vi "Example 2.vi"() -> ()   [LabVIEW 2019]
uses:
  FINS/FINS_header.ctl
  subvi/Request.ctl
  FINS/FINS CMD.ctl
  FINS/FINS TCP.lvlib
panel:
  out "error":string
  out "CMD":T1
  out "FINS Header Sever":T2={"resp req"=FALSE, "cmd resp"=FALSE, "SID"=255, "DNA"=2, "DA1"=2, "DA2"=2, "SA1"=0, "SA2"=255, "SNA"=255} {"SNA" max=127 format="%x"; "SA2" max=254 step=1 format="%x"; "SA1" format="%x"; "DA2" max=254 step=1 format="%x"; "DA1" format="%x"; "DNA" max=127 step=1 format="%x"}
  out "error TCP out":errorcluster={"status"=TRUE, "code"=56, "source"="TCP Read in main.vi"}
  in  "Request":T3=enum."Read_002"
  out "RSP":bool
  in  "Acces Release":bool
  in  "Acces Acq":bool
  out "t2":dbl
  out "t1":dbl
  out "Client Node":u32=10 format="%x"
  in  "FINS Header Client":T2={"resp req"=TRUE, "cmd resp"=FALSE, "SID"=0, "DNA"=0, "DA1"=10, "DA2"=0, "SA1"=0, "SA2"=251, "SNA"=0} {"SNA" max=127 format="%x"; "SA2" max=254 step=1 format="%x"; "SA1" format="%x"; "DA2" max=254 step=1 format="%x"; "DA1" format="%x"; "DNA" max=127 step=1 format="%x"}
  in  "send request":bool
  out "count":i32=1
  out "Server Node":u32=10 format="%x"
  out "cmd":u32=1
  out "error TCP in":errorcluster={"status"=TRUE, "code"=56, "source"="TCP Read in main.vi"}
  in  "setup":bool
  out "len":i32=24
  out "on":bool
  out "data out":string
  in  "stop":bool=TRUE
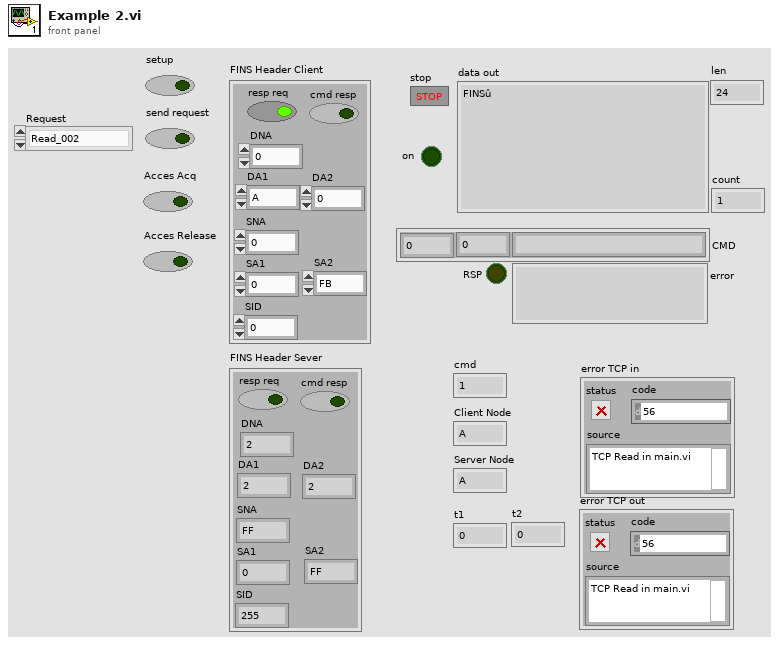
[diagram p1: front panel]
types:
  T1 = typedef "FINS TCP.lvlib/FINS CMD.ctl" = cluster{"MR":u8, "SR":u8, "name":string}
  T2 = typedef "FINS TCP.lvlib/FINS_header.ctl" = cluster{"resp req":bool, "cmd resp":bool, "SID":u8, "DNA":u8, "DA1":u8, "DA2":u8, "SA1":u8, "SA2":u8, "SNA":u8}
  T3 = typedef "Request.ctl" = enum16{"Setup", "Access Right: Acquire", "Access Right: Release", "STOP", "RUN", "Read_001", "Read_002", "Read_003", "Write_001"}
  T4 = enum16{"Standard", "Buffered", "CRLF", "Immediate"}
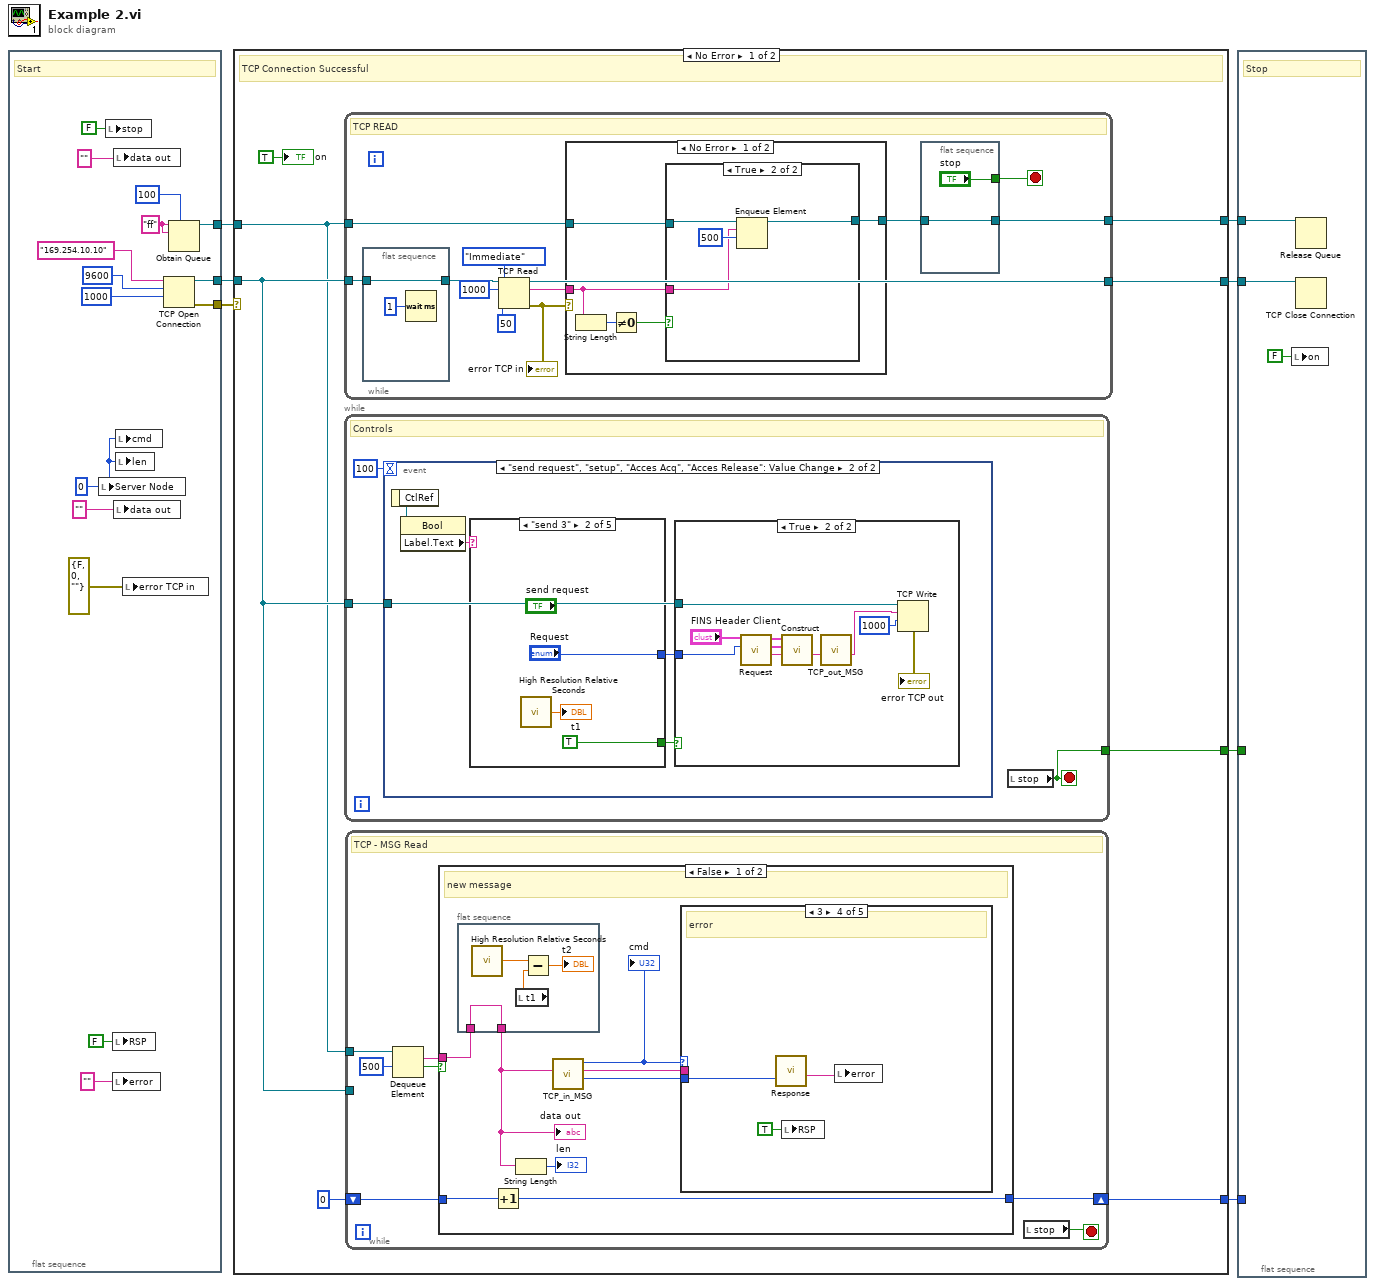
[diagram p0: block diagram]
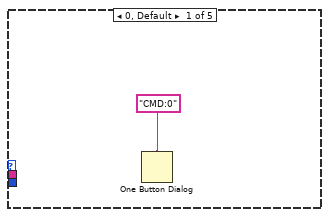
[diagram p2: hidden frame]
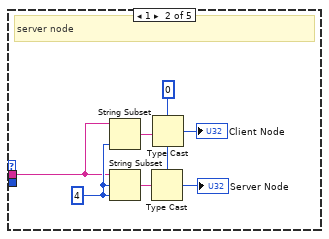
[diagram p3: hidden frame]
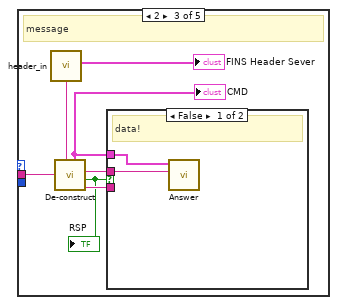
[diagram p4: hidden frame]
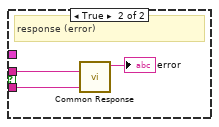
[diagram p5: hidden frame]
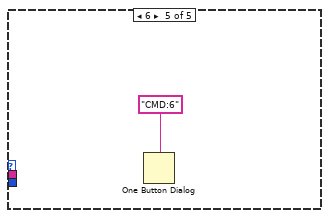
[diagram p6: hidden frame]
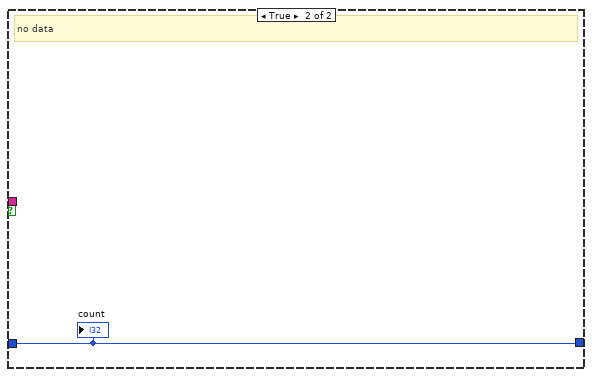
[diagram p7: hidden frame]
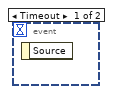
[diagram p8: hidden frame]
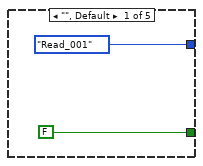
[diagram p10: hidden frame]
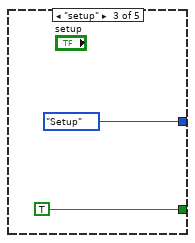
[diagram p11: hidden frame]
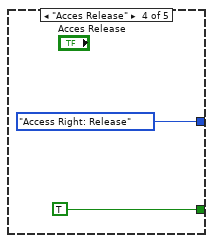
[diagram p12: hidden frame]
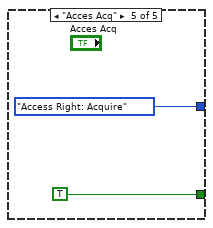
[diagram p13: hidden frame]
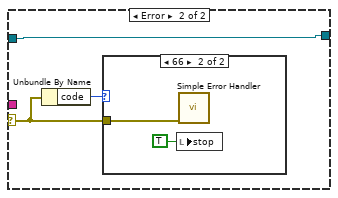
[diagram p15: hidden frame]
diagram:
  n1 = flat-sequence {
    tunnel: [w19] -> w7
    tunnel: [w18] -> w6
    tunnel: [w13] -> w3
    frame #0 {
      w12 = u32 0 ("snode")
      w14 = "ff" ("name (unnamed)")
      # "Start"
      n2 = local write "Server Node"(w12) -> ()
      n3 = local write "stop"(FALSE ("stop")) -> ()
      n4 = local write "RSP"(FALSE ("RSP")) -> ()
      n5 = local write "error"("" ("message")) -> ()
      n6 = local write "data out"("" ("data out")) -> ()
      n7 = local write "data out"("" ("data out")) -> ()
      n8 = local write "cmd"(w12) -> ()
      n9 = local write "len"(w12) -> ()
      n10 = local write "error TCP in"(errorcluster {"status"=FALSE, "code"=0, "source"=""} ("error out")) -> ()
      n11 = TCP Open Connection(address="169.254.10.10", remote port or service name=u16 9600, timeout ms (60000)=1000) -> (connection ID=w19:refnum<k5>, error out=w18:errorcluster)  [unwired: 2 in]
      n12 = Obtain Queue(max queue size (-1, unlimited)=100, name (unnamed)=w14, element data type=w14) -> (queue out=w13:refnum<queue>)  [unwired: 2 in, 2 out]
    }
  }
  n13 = case shown="No Error" w6 {
    tunnel: w7 -> [w28 w136]
    tunnel: [w29 w136] -> w5
    tunnel: [w27 w135] -> w4
    tunnel: w3 -> [w26 w135]
    tunnel: [w24 _] -> w2
    tunnel: [w23 _] -> w1
    frame No Error {
      # "TCP Connection Successful"
      n14 = while {
        tunnel: w28 -> [w110]
        tunnel: [w114] -> w29
        tunnel: w26 -> [w107]
        tunnel: [w106] -> w27
        stop <- w104 stop-if-true
        # "TCP READ"
        n15 = flat-sequence {
          tunnel: [w119] -> w111
          tunnel: w110 -> [w119]
          frame #0 {
            n16 = Wait (ms)(milliseconds to wait=u32 1) -> ()  [unwired: 1 out]
          }
        }
        n17 = TCP Read(connection ID=w111, bytes to read=1000, 7:T4."Immediate" ("mode (standard)"), 9:50 ("timeout ms (25000)")) -> (connection ID out=w114:refnum<k5>, data out=w112:string, error out=w113:errorcluster)  [unwired: 1 in]
        "error TCP in" <- w113
        n18 = case shown="No Error" w113 {
          selector: w113 -> [_ w130]
          tunnel: w112 -> [w122 _]
          tunnel: w107 -> [w121 w132]
          tunnel: [w120 w132] -> w105
          frame No Error {
            n19 = String Length(string=w122) -> (length=w124:i32)
            n20 = Not Equal To 0?(x=w124) -> (x != 0?=w123:bool)
            n21 = case shown="True" w123 {
              tunnel: w122 -> [_ w126]
              tunnel: w121 -> [w125 w128]
              tunnel: [w125 w127] -> w120
              frame False {
              }
              frame True {
                n22 = Enqueue Element(queue=w128, element=w126, timeout in ms (-1)=500) -> (queue out=w127:refnum<queue>)  [unwired: 1 in, 2 out]
              }
            }
          }
          frame Error {
            n23 = Unbundle By Name(w130) -> ("code"=w131:i32)
            n24 = case shown="66" w131 {
              tunnel: w130 -> [_ w134]
              frame 0, Default {
              }
              frame 66 {
                n25 = local write "stop"(TRUE ("stop")) -> ()
                n26 = call <vilib>:"Simple Error Handler.vi"("error in (no error)"=w134) -> ()  [unwired: 4 in, 5 out]
              }
            }
          }
        }
        n27 = flat-sequence {
          tunnel: [w117] -> w106
          tunnel: w105 -> [w117]
          tunnel: ["stop"] -> w104
          frame #0 {
          }
        }
      }
      n28 = while {
        tunnel: w28 -> [w76]
        tunnel: [w75] -> w23
        stop <- w75 stop-if-true
        # "Controls"
        n29 = event shown="[1] \"send request\", \"setup\", \"Acces Acq\", \"Acces Release\": Value Change" {
          selector: _ -> [_ _]
          dyn-events: _ -> [_ _]
          timeout: 100 -> [_ _]
          tunnel: w76 -> [_ w79]
          event Timeout {
            n30 = event-data() -> ()  [unwired: 1 in, 1 out]
          }
          event "send request", "setup", "Acces Acq", "Acces Release": Value Change {
            n31 = event-data() -> ("CtlRef"=w82:refnum<vi>)  [unwired: 1 in]
            n32 = property class="Bool"(reference=w82) -> ("Label.Text"=w81:string)  [unwired: 1 in, 2 out]
            n33 = case shown="\"send 3\"" w81 {
              tunnel: [FALSE TRUE TRUE TRUE TRUE] -> w80
              tunnel: [Request."Read_001" ("Request") "Request" Request."Setup" ("Request") Request."Access Right: Release" ("Request") Request."Access Right: Acquire" ("Request")] -> w78
              frame "", Default {
              }
              frame "send 3" {
                n34 = call <vilib>:"High Resolution Relative Seconds.vi"() -> ("relative seconds"=→"t1":dbl)
              }
              frame "setup" {
              }
              frame "Acces Release" {
              }
              frame "Acces Acq" {
              }
            }
            n35 = case shown="True" w80 {
              tunnel: w79 -> [_ w91]
              tunnel: w78 -> [_ w86]
              frame False {
              }
              frame True {
                n36 = call "Request.vi"("Request"=w86, "FINS Header i"="FINS Header Client") -> ("Paramters"=w83:string, "FINS CMD"=w84:T1, "FINS Header o"=w85:T2)  [unwired: 6 in, 1 out]
                n37 = call "Construct.vi"("Paramters"=w83, "FINS CMD"=w84, "FINS Header"=w85) -> ("msg"=w90:string)  [unwired: 8 in]
                n38 = call "TCP_out_MSG.vi"("msgin"=w90) -> ("msg"=w89:string)  [unwired: 10 in]
                n39 = TCP Write(connection ID=w91, data in=w89, 9:1000 ("timeout ms (25000)")) -> (error out=→"error TCP out":errorcluster)  [unwired: 1 in, 2 out]
              }
            }
          }
        }
        n40 = local read "stop"() -> (w75:bool)
      }
      n41 = while {
        tunnel: w28 -> [_]
        tunnel: w26 -> [w36]
        shift-right: [w31] -> w24
        shift-left: 0 -> [w32]
        stop <- w37 stop-if-true
        # "TCP - MSG Read"
        n42 = Dequeue Element(queue=w36, timeout in ms (-1)=500) -> (element=w33:string, timed out?=w34:bool)  [unwired: 1 in, 2 out]
        n43 = case shown="False" w34 {
          tunnel: w33 -> [w39 _]
          tunnel: w32 -> [w42 w74]
          tunnel: [w41 w74] -> w31
          frame False {
            # "new message"
            n44 = flat-sequence {
              tunnel: [w73] -> w40
              tunnel: w39 -> [w73]
              frame #0 {
                n45 = call <vilib>:"High Resolution Relative Seconds.vi"() -> ("relative seconds"=w72:dbl)
                n46 = local read "t1"() -> (w71:dbl)
                n47 = Subtract(x=w72, y=w71) -> (x-y=→"t2":dbl)
              }
            }
            n48 = Increment(x=w42) -> (x+1=w41:i32)
            n49 = String Length(string=w40) -> (length=→"len":i32)
            n50 = call "TCP_in_MSG.vi"("msg i"=w40) -> ("rsp"=w38:u32, "msg o"=w43:string, "cmd"=w44:u32)  [unwired: 8 in]
            "cmd" <- w44
            n51 = case shown="3" w44 {
              tunnel: w43 -> [_ w51 w60 _ _]
              tunnel: w38 -> [_ _ _ w68 _]
              frame 0, Default {
                n52 = One Button Dialog(message="CMD:0") -> ()  [unwired: 1 in, 1 out]
              }
              frame 1 {
                w49 = u32 0 ("length")
                w52 = 4 ("length (rest)")
                # "server node"
                n53 = String Subset(string=w51, length (rest)=w52) -> (substring=w50:string)  [unwired: 1 in]
                n54 = String Subset(string=w51, offset (0)=w52, length (rest)=w52) -> (substring=w53:string)
                n55 = Type Cast(type=w49, x=w53) -> (*(type *) &x=→"Server Node":u32)
                n56 = Type Cast(type=w49, x=w50) -> (*(type *) &x=→"Client Node":u32)
              }
              frame 2 {
                # "message"
                n57 = call "De-construct.vi"("msg o"=w60) -> ("MSES/SRES"=w59:string, "RSP?"=w56:bool, "Data"=w57:string, "CMD"=w55:T1, "header"=w58:string)  [unwired: 6 in]
                "CMD" <- w55
                "RSP" <- w56
                n58 = call "header_in.vi"("HEADER"=w58) -> ("FINS Header"=→"FINS Header Sever":T2)  [unwired: 10 in]
                n59 = case shown="False" w56 {
                  tunnel: w59 -> [_ w64]
                  tunnel: w57 -> [w61 w65]
                  tunnel: w55 -> [w62 _]
                  frame False {
                    # "data!"
                    n60 = call "Answer.vi"("Data"=w61, "CMD 2"=w62) -> ()  [unwired: 8 in, 2 out]
                  }
                  frame True {
                    # "response (error)"
                    n61 = call "Common Response.vi"("RSP"=w64, "Data"=w65) -> ("error"=→"error":string)  [unwired: 6 in, 3 out]
                  }
                }
              }
              frame 3 {
                # "error"
                n62 = call "Response.vi"("rsp"=w68) -> ("error"=w66:string)  [unwired: 10 in]
                n63 = local write "RSP"(TRUE ("RSP")) -> ()
                n64 = local write "error"(w66) -> ()
              }
              frame 6 {
                n65 = One Button Dialog(message="CMD:6") -> ()  [unwired: 1 in, 1 out]
              }
            }
            "data out" <- w40
          }
          frame True {
            # "no data"
            "count" <- w74
          }
        }
        n66 = local read "stop"() -> (w37:bool)
      }
      "on" <- TRUE
    }
    frame Error {
      # "TCP Connection Error"
    }
  }
  n67 = flat-sequence {
    tunnel: w5 -> [w139]
    tunnel: w4 -> [w137]
    tunnel: w2 -> [_]
    tunnel: w1 -> [_]
    frame #0 {
      # "Stop"
      n68 = local write "on"(FALSE ("on")) -> ()
      n69 = Release Queue(queue=w137) -> ()  [unwired: 2 in, 3 out]
      n70 = TCP Close Connection(connection ID=w139) -> ()  [unwired: 2 in, 2 out]
    }
  }
